vi "Acme Calculator.vi"() -> ()   [LabVIEW 2014]
doc: "This is an example top-level VI that will be built into an EXE."
uses:
  mymathlib/acme_math.lvlib
panel:
  out "Result":dbl
  in  "Y":dbl
  in  "X":dbl
  in  "Divide":bool
  in  "Multiply":bool
  in  "Subtract":bool
  in  "Add":bool
  # "Choose Operation"
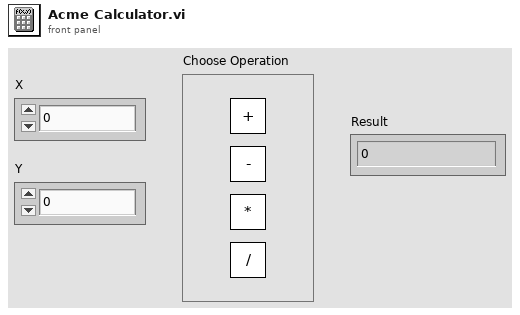
[diagram p1: front panel]
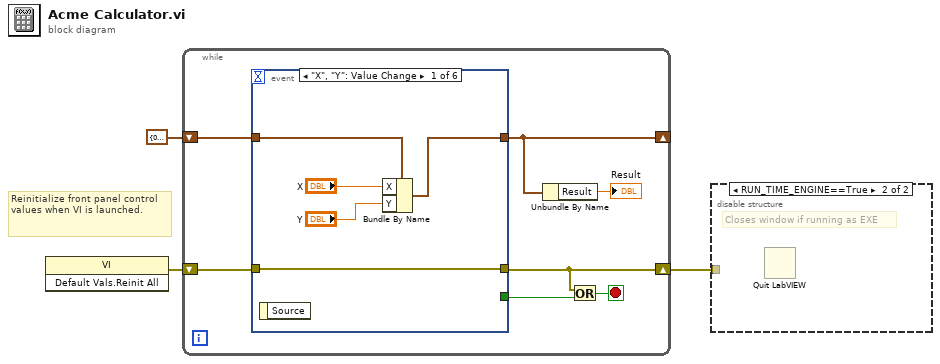
[diagram p0: block diagram]
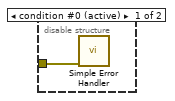
[diagram p2: hidden frame]
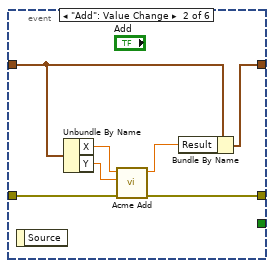
[diagram p3: hidden frame]
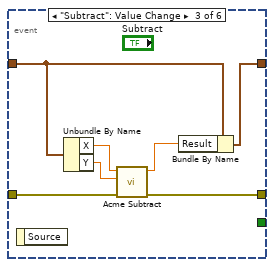
[diagram p4: hidden frame]
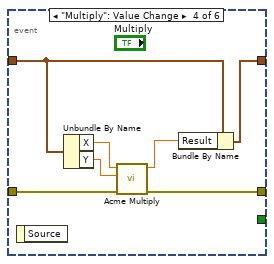
[diagram p5: hidden frame]
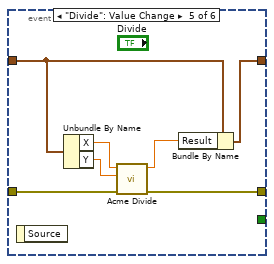
[diagram p6: hidden frame]
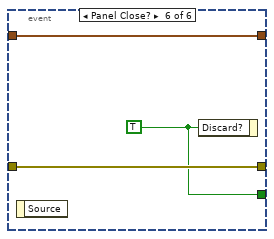
[diagram p7: hidden frame]
diagram:
  # "Reinitialize front panel control values when VI is launched."
  n1 = invoke class="VI" method="Default Vals.Reinit All"() -> (error out=w1:errorcluster)  [unwired: 3 in, 2 out]
  n2 = while {
    shift-right: [w6] -> w3
    shift-left: w1 -> [w10]
    shift-right: [w8] -> _
    shift-left: cluster{"X":dbl, "Y":dbl, "Result":dbl} {"X"=0.0, "Y"=0.0, "Result"=0.0} -> [w9]
    stop <- w4 stop-if-true
    n3 = event shown="[0] \"X\", \"Y\": Value Change" {
      selector: _ -> [_ _ _ _ _ _]
      dyn-events: _ -> [_ _ _ _ _ _]
      timeout: _ -> [_ _ _ _ _ _]
      tunnel: w10 -> [w11 w22 w29 w36 w43 w46]
      tunnel: [w11 w21 w28 w35 w42 w46] -> w6
      tunnel: [_ _ _ _ _ w45] -> w5
      tunnel: w9 -> [w15 w18 w25 w32 w39 w44]
      tunnel: [w12 w17 w24 w31 w38 w44] -> w8
      event "X", "Y": Value Change {
        n4 = event-data() -> ()  [unwired: 1 in, 1 out]
        n5 = Bundle By Name(cluster=w15, "X"="X", "Y"="Y") -> (w12:cluster{"X":dbl, "Y":dbl, "Result":dbl})
      }
      event "Add": Value Change {
        n6 = event-data() -> ()  [unwired: 1 in, 1 out]
        n7 = Unbundle By Name(w18) -> ("X"=w20:dbl, "Y"=w19:dbl)
        n8 = call "Acme Add.vi"("error in (no error)"=w22, "y"=w19, "x"=w20) -> ("error out"=w21:errorcluster, "sum"=w16:dbl)  [unwired: 7 in]
        n9 = Bundle By Name(cluster=w18, "Result"=w16) -> (w17:cluster{"X":dbl, "Y":dbl, "Result":dbl})
      }
      event "Subtract": Value Change {
        n10 = event-data() -> ()  [unwired: 1 in, 1 out]
        n11 = Unbundle By Name(w25) -> ("X"=w27:dbl, "Y"=w26:dbl)
        n12 = call "Acme Subtract.vi"("error in (no error)"=w29, "y"=w26, "x"=w27) -> ("error out"=w28:errorcluster, "difference"=w23:dbl)  [unwired: 7 in]
        n13 = Bundle By Name(cluster=w25, "Result"=w23) -> (w24:cluster{"X":dbl, "Y":dbl, "Result":dbl})
      }
      event "Multiply": Value Change {
        n14 = event-data() -> ()  [unwired: 1 in, 1 out]
        n15 = Unbundle By Name(w32) -> ("X"=w34:dbl, "Y"=w33:dbl)
        n16 = call "Acme Multiply.vi"("error in (no error)"=w36, "y"=w33, "x"=w34) -> ("error out"=w35:errorcluster, "product"=w30:dbl)  [unwired: 7 in]
        n17 = Bundle By Name(cluster=w32, "Result"=w30) -> (w31:cluster{"X":dbl, "Y":dbl, "Result":dbl})
      }
      event "Divide": Value Change {
        n18 = event-data() -> ()  [unwired: 1 in, 1 out]
        n19 = Unbundle By Name(w39) -> ("X"=w41:dbl, "Y"=w40:dbl)
        n20 = call "Acme Divide.vi"("error in (no error)"=w43, "y"=w40, "x"=w41) -> ("error out"=w42:errorcluster, "x/y"=w37:dbl)  [unwired: 7 in]
        n21 = Bundle By Name(cluster=w39, "Result"=w37) -> (w38:cluster{"X":dbl, "Y":dbl, "Result":dbl})
      }
      event Panel Close? {
        w45 = TRUE ("Discard?")
        n22 = event-data() -> ()  [unwired: 1 in, 1 out]
        n23 = event-data("Discard?"=w45) -> ()  [unwired: 1 in, 1 out]
      }
    }
    n24 = Unbundle By Name(w8) -> ("Result"=→"Result":dbl)
    n25 = Or(x=w6, y=w5) -> (x .or. y?=w4:bool)
  }
  n26 = disable-structure shown="RUN_TIME_ENGINE==True" {
    disable-tunnel: w3 -> [w47 _]
    frame condition #0 (active) {
      n27 = call <vilib>:"Simple Error Handler.vi"("error in (no error)"=w47) -> ()  [unwired: 4 in, 5 out]
    }
    frame condition #1 {
      # "Closes window if running as EXE"
      n28 = Quit LabVIEW() -> ()  [unwired: 1 in]
    }
  }
